vi "SchreibeWegzähler.vi"(8 "error in (no error)":errorcluster caption="Fehler (Eingang, kein Fehler)", 11 "Aktuell":dbl) -> (0 "error out":errorcluster caption="Fehler (Ausgang)")   [LabVIEW 2014]
uses:
  <vilib>/Utility/config.llb/Read Key (Double).vi
  <vilib>/Utility/config.llb/Write Key (Double).vi
  <vilib>/Utility/config.llb/NI_LVConfig.lvlib
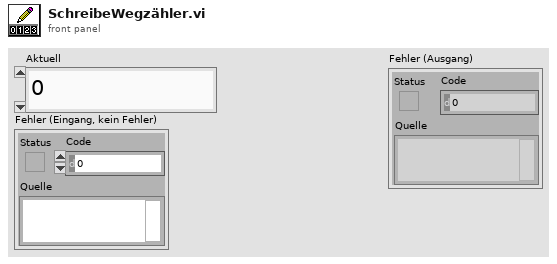
[diagram p1: front panel]
types:
  T1 = typedef "NI_LVConfig.lvlib/Config Data RefNum.ctl" = refnum<k1>
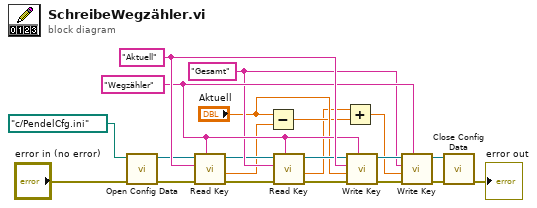
[diagram p0: block diagram]
diagram:
  w9 = "Gesamt" ("key")
  w17 = "Aktuell" ("key")
  w10 = "Wegzähler" ("section")
  n1 = call <vilib>:"Open Config Data.vi"("error in (no error)"="error in (no error)", "configuration file path"=path "c:/PendelCfg.ini") -> ("error out"=w2:errorcluster, "refnum"=w16:T1)  [unwired: 7 in, 1 out]
  n2 = call-poly <vilib>:"Read Key.vi"("section"=w10, "error in (no error)"=w2, "key"=w17, "refnum"=w16) -> ("error out"=w18:errorcluster, "value"=w7:dbl, "refnum out"=w8:T1)  [unwired: 4 in, 1 out]
  n3 = Subtract(x="Aktuell", y=w7) -> (x-y=w5:dbl)
  n4 = call-poly <vilib>:"Read Key.vi"("section"=w10, "error in (no error)"=w18, "key"=w9, "refnum"=w8) -> ("error out"=w1:errorcluster, "value"=w4:dbl, "refnum out"=w15:T1)  [unwired: 4 in, 1 out]
  n5 = Add(x=w4, y=w5) -> (x+y=w3:dbl)
  n6 = call-poly <vilib>:"Write Key.vi"("section"=w10, "error in (no error)"=w1, "value"="Aktuell", "key"=w17, "refnum"=w15) -> ("error out"=w13:errorcluster, "refnum out"=w14:T1)  [unwired: 4 in, 1 out]
  n7 = call-poly <vilib>:"Write Key.vi"("section"=w10, "error in (no error)"=w13, "value"=w3, "key"=w9, "refnum"=w14) -> ("error out"=w12:errorcluster, "refnum out"=w11:T1)  [unwired: 4 in, 1 out]
  n8 = call <vilib>:"Close Config Data.vi"("error in (no error)"=w12, "refnum"=w11) -> ("error out"=→"error out":errorcluster)  [unwired: 8 in, 1 out]
